vi "bmp get temperature c.vi"(8 "error in (no error)":errorcluster) -> (0 "error out":errorcluster, 3 "function return":sgl)   [LabVIEW 2014, in "libroboticscape.lvlib"]
doc: "float bmp_get_temperature_c();"
uses:
  libroboticscape.lvlib
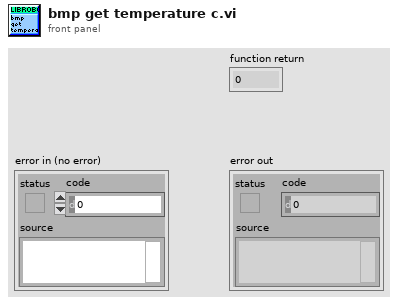
[diagram p1: front panel]
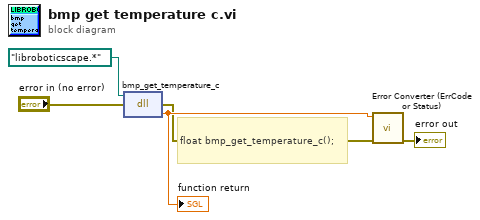
[diagram p0: block diagram]
diagram:
  # "float bmp_get_temperature_c();"
  n1 = dll-call lib="C:/Users/ktalke/Documents/Robotics-Cape-Master-Jessie/Libroboticscape-Master-Jessie/libroboticscape.so" fn="bmp_get_temperature_c"(path in=path "libroboticscape.*", error in="error in (no error)") -> (error out=w3:errorcluster, "return type"=w5:sgl)  [unwired: 1 in, 1 out]
  "function return" <- w5
  n2 = call "Error Converter (ErrCode or Status).vi"("error in (no error)"=w3, "error code"=w5) -> ("error out"=→"error out":errorcluster)  [unwired: 9 in]
